vi "GFITS_toInternalDHSFits.vi"(3 "nodeID":string, 4 "ms timeout (-1)":i32=-1, 5 "response Q":string, 6 "key":string, 7 "error in (no error)":errorcluster, 11 "command":string) -> (0 "error out":errorcluster, 1 "response":errorcluster)   [LabVIEW 2016]
panel:
  in  "cmd struct":T1
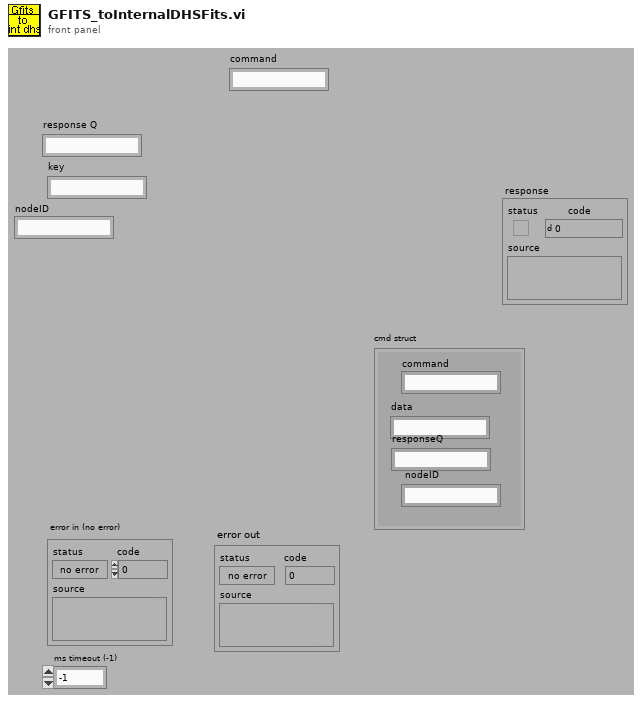
[diagram p1: front panel]
types:
  T1 = cluster{"command":string, "data":string, "responseQ":string, " nodeID":string}
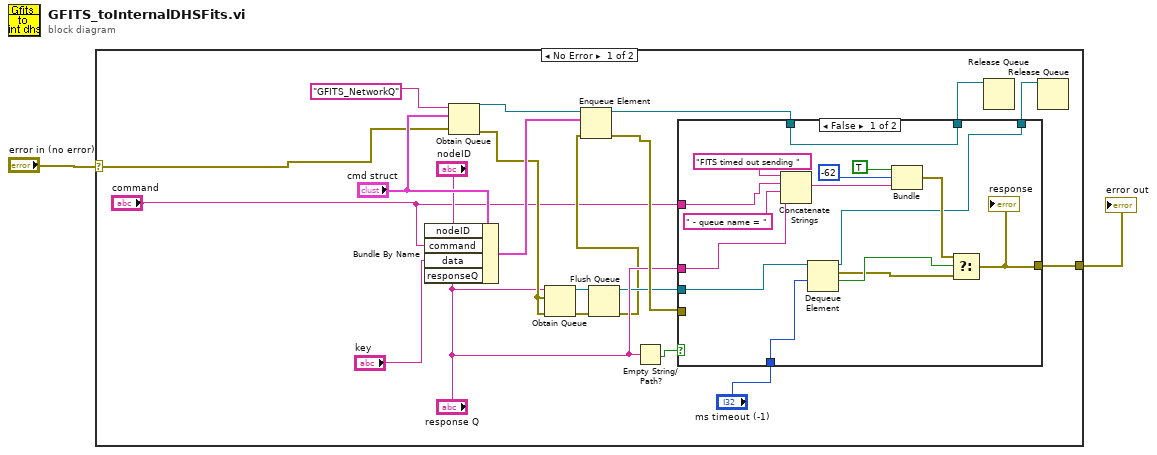
[diagram p0: block diagram]
diagram:
  n1 = case shown="No Error" "error in (no error)" {
    selector: "error in (no error)" -> [w16 w42]
    tunnel: [w20 w42] -> w1
    frame No Error {
      n2 = Bundle By Name(cluster="cmd struct", "nodeID"="nodeID", "command"="command", "data"="key", "responseQ"="response Q") -> (w17:T1)
      n3 = Obtain Queue(name (unnamed)="GFITS_NetworkQ", element data type="cmd struct", error in (no error)=w16) -> (queue out=w18:refnum<queue>, error out=w12:errorcluster)  [unwired: 2 in, 1 out]
      n4 = Obtain Queue(name (unnamed)="response Q", element data type=w12, error in (no error)=w12) -> (queue out=w9:refnum<queue>, error out=w8:errorcluster)  [unwired: 2 in, 1 out]
      n5 = Flush Queue(queue=w9, error in (no error)=w8) -> (queue out=w7:refnum<queue>, error out=w6:errorcluster)  [unwired: 1 out]
      n6 = Enqueue Element(queue=w18, element=w17, error in (no error)=w6) -> (queue out=w14:refnum<queue>, error out=w13:errorcluster)  [unwired: 2 out]
      n7 = Empty String/Path?(string/path="response Q") -> (empty?=w22:bool)
      n8 = case shown="False" w22 {
        tunnel: "response Q" -> [w30 _]
        tunnel: "ms timeout (-1)" -> [w27 _]
        tunnel: w13 -> [_ w41]
        tunnel: [w38 w41] -> w20
        tunnel: "command" -> [w37 _]
        tunnel: [w26 w40] -> w15
        tunnel: w14 -> [w26 w40]
        tunnel: w7 -> [w25 w39]
        tunnel: [w24 w39] -> w11
        frame False {
          n9 = Concatenate Strings("FITS timed out sending " ("source"), w37, " - queue name = ", w30) -> (w34:string)
          n10 = Dequeue Element(queue=w25, timeout in ms (-1)=w27) -> (queue out=w24:refnum<queue>, element=w28:errorcluster, timed out?=w29:bool)  [unwired: 1 in, 1 out]
          n11 = Bundle(TRUE, -62, w34) -> (w35:errorcluster)  [unwired: 1 out]
          n12 = Select(t=w35, s=w29, f=w28) -> (s? t:f=w38:errorcluster)
          "response" <- w38
        }
        frame True {
        }
      }
      n13 = Release Queue(queue=w15) -> ()  [unwired: 1 in, 4 out]
      n14 = Release Queue(queue=w11) -> ()  [unwired: 1 in, 4 out]
    }
    frame Error {
    }
  }
  "error out" <- w1
